vi "Init Data Object.vi"(11 "Data in":refnum<class "Data.lvclass">) -> (3 "Data out":refnum<class "Data.lvclass">)   [LabVIEW 2014, in "Base Data Class.lvlib" / "Data.lvclass"]
uses:
  Data.lvclass
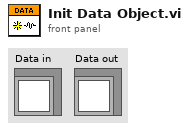
[diagram p1: front panel]
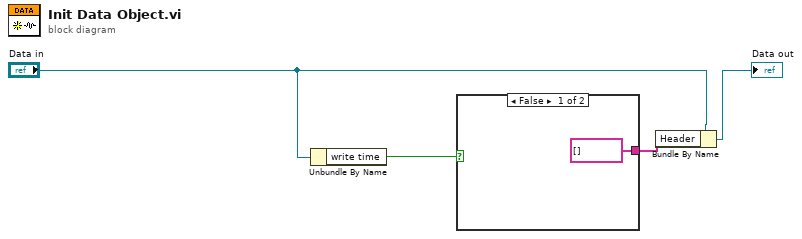
[diagram p0: block diagram]
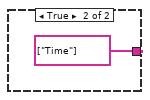
[diagram p2: hidden frame]
diagram:
  n1 = Unbundle By Name("Data in") -> ("write time"=w2:bool)
  n2 = case shown="False" w2 {
    tunnel: [string[] [] string[] ["Time"]] -> w1
    frame False {
    }
    frame True {
    }
  }
  n3 = Bundle By Name(cluster="Data in", "Header"=w1) -> (→"Data out":refnum<class "Data.lvclass">)
